vi "RichToFlatnixnet_grpc_ReadStateValue.vi"(5 "OutputClusterType":T1, 11 "InputCluster":T14) -> (3 "OutputCluster":T1)   [LabVIEW 2025, in "xnet-grpc_client.lvlib"]
uses:
  nixnet_grpc_ReadStateValue.ctl
  nixnet_grpc_ReadStateValue_value/nixnet_grpc_ReadStateValue_value.lvclass
  nixnet_grpc_ReadStateValue_Flat.ctl
  nixnet_grpc_CanCommResponse_Flat.ctl
  nixnet_grpc_CanCommState.ctl
  nixnet_grpc_CanLastErr.ctl
  nixnet_grpc_FlexRayCommResponse_Flat.ctl
  nixnet_grpc_FlexRayPocState.ctl
  nixnet_grpc_FlexRayStats_Flat.ctl
  nixnet_grpc_LinCommResponse_Flat.ctl
  nixnet_grpc_LinCommState.ctl
  nixnet_grpc_SessionInfoResponse_Flat.ctl
  nixnet_grpc_SessionInfoState.ctl
  nixnet_grpc_J1939CommState_Flat.ctl
  nixnet_grpc_TimeLocalNetwork_Flat.ctl
  xnet-grpc_client.lvlib
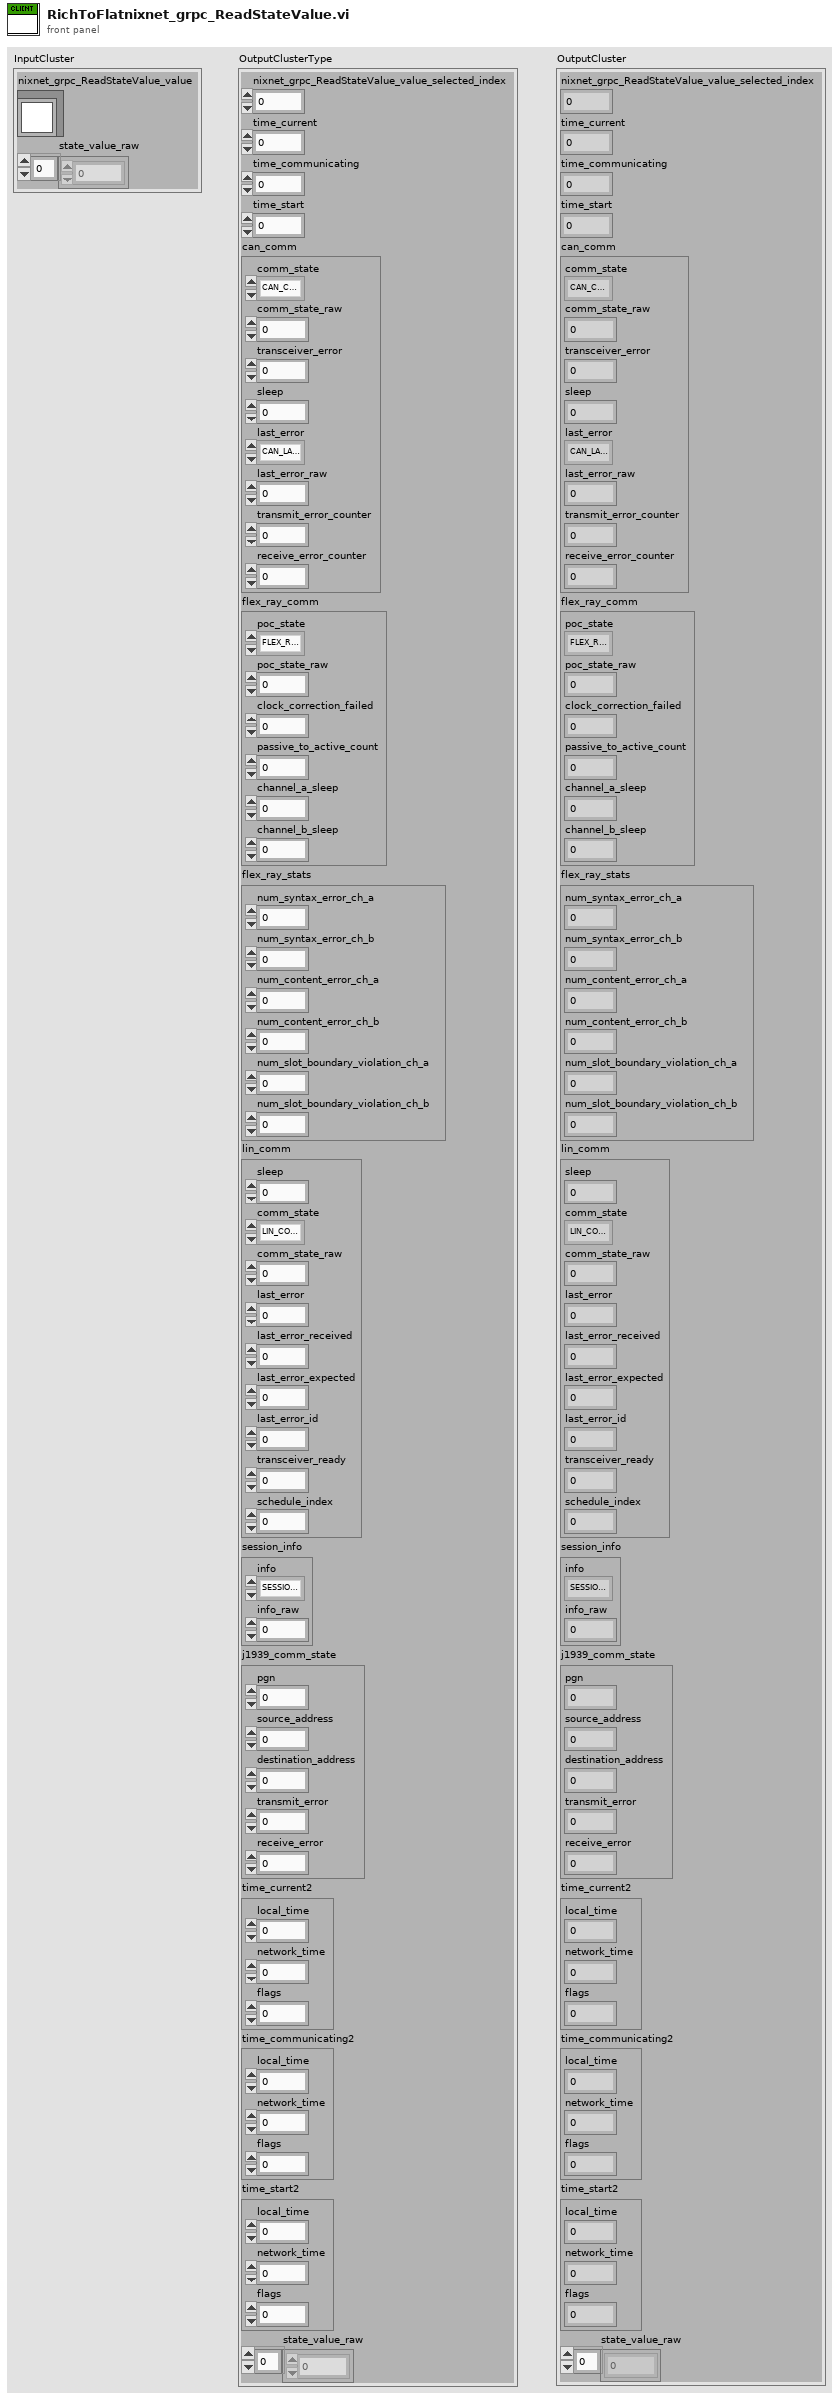
[diagram p1: front panel]
types:
  T1 = typedef "xnet-grpc_client.lvlib/nixnet_grpc_ReadStateValue_Flat.ctl" = cluster{"nixnet_grpc_ReadStateValue_value_selected_index":i32, "time_current":u64, "time_communicating":u64, "time_start":u64, "can_comm":T2, "flex_ray_comm":T5, "flex_ray_stats":T7, "lin_comm":T8, "session_info":T10, "j1939_comm_state":T12, "time_current2":T13, "time_communicating2":T13, "time_start2":T13, "state_value_raw":u8[]}
  T2 = typedef "xnet-grpc_client.lvlib/nixnet_grpc_CanCommResponse_Flat.ctl" = cluster{"comm_state":T3, "comm_state_raw":u32, "transceiver_error":u32, "sleep":u32, "last_error":T4, "last_error_raw":u32, "transmit_error_counter":u32, "receive_error_counter":u32}
  T3 = typedef "xnet-grpc_client.lvlib/nixnet_grpc_CanCommState.ctl" = enum32{"CAN_COMM_STATE_ERROR_ACTIVE", "CAN_COMM_STATE_ERROR_PASSIVE", "CAN_COMM_STATE_BUS_OFF", "CAN_COMM_STATE_INIT"}
  T4 = typedef "xnet-grpc_client.lvlib/nixnet_grpc_CanLastErr.ctl" = enum32{"CAN_LAST_ERR_NONE", "CAN_LAST_ERR_STUFF", "CAN_LAST_ERR_FORM", "CAN_LAST_ERR_ACK", "CAN_LAST_ERR_BIT_1", "CAN_LAST_ERR_BIT_0", "CAN_LAST_ERR_CRC"}
  T5 = typedef "xnet-grpc_client.lvlib/nixnet_grpc_FlexRayCommResponse_Flat.ctl" = cluster{"poc_state":T6, "poc_state_raw":u32, "clock_correction_failed":u32, "passive_to_active_count":u32, "channel_a_sleep":u32, "channel_b_sleep":u32}
  T6 = typedef "xnet-grpc_client.lvlib/nixnet_grpc_FlexRayPocState.ctl" = enum32{"FLEX_RAY_POC_STATE_DEFAULT_CONFIG", "FLEX_RAY_POC_STATE_READY", "FLEX_RAY_POC_STATE_NORMAL_ACTIVE", "FLEX_RAY_POC_STATE_NORMAL_PASSIVE", "FLEX_RAY_POC_STATE_HALT", "FLEX_RAY_POC_STATE_MONITOR", "FLEX_RAY_POC_STATE_CONFIG"}
  T7 = typedef "xnet-grpc_client.lvlib/nixnet_grpc_FlexRayStats_Flat.ctl" = cluster{"num_syntax_error_ch_a":u32, "num_syntax_error_ch_b":u32, "num_content_error_ch_a":u32, "num_content_error_ch_b":u32, "num_slot_boundary_violation_ch_a":u32, "num_slot_boundary_violation_ch_b":u32}
  T8 = typedef "xnet-grpc_client.lvlib/nixnet_grpc_LinCommResponse_Flat.ctl" = cluster{"sleep":u32, "comm_state":T9, "comm_state_raw":u32, "last_error":u32, "last_error_received":u32, "last_error_expected":u32, "last_error_id":u32, "transceiver_ready":u32, "schedule_index":u32}
  T9 = typedef "xnet-grpc_client.lvlib/nixnet_grpc_LinCommState.ctl" = enum32{"LIN_COMM_STATE_IDLE", "LIN_COMM_STATE_ACTIVE", "LIN_COMM_STATE_INACTIVE"}
  T10 = typedef "xnet-grpc_client.lvlib/nixnet_grpc_SessionInfoResponse_Flat.ctl" = cluster{"info":T11, "info_raw":u32}
  T11 = typedef "xnet-grpc_client.lvlib/nixnet_grpc_SessionInfoState.ctl" = enum32{"SESSION_INFO_STATE_STOPPED", "SESSION_INFO_STATE_STARTED", "SESSION_INFO_STATE_MIX"}
  T12 = typedef "xnet-grpc_client.lvlib/nixnet_grpc_J1939CommState_Flat.ctl" = cluster{"pgn":u32, "source_address":u32, "destination_address":u32, "transmit_error":u32, "receive_error":u32}
  T13 = typedef "xnet-grpc_client.lvlib/nixnet_grpc_TimeLocalNetwork_Flat.ctl" = cluster{"local_time":u64, "network_time":u64, "flags":u32}
  T14 = typedef "xnet-grpc_client.lvlib/nixnet_grpc_ReadStateValue.ctl" = cluster{"nixnet_grpc_ReadStateValue_value":refnum<class "nixnet_grpc_ReadStateValue_value.lvclass">, "state_value_raw":u8[]}
  T15 = typedef "xnet-grpc_client.lvlib/nixnet_grpc_CanCommResponse.ctl" = cluster{"comm_state":T3, "comm_state_raw":u32, "transceiver_error":u32, "sleep":u32, "last_error":T4, "last_error_raw":u32, "transmit_error_counter":u32, "receive_error_counter":u32}
  T16 = typedef "xnet-grpc_client.lvlib/nixnet_grpc_FlexRayCommResponse.ctl" = cluster{"poc_state":T6, "poc_state_raw":u32, "clock_correction_failed":u32, "passive_to_active_count":u32, "channel_a_sleep":u32, "channel_b_sleep":u32}
  T17 = typedef "xnet-grpc_client.lvlib/nixnet_grpc_FlexRayStats.ctl" = cluster{"num_syntax_error_ch_a":u32, "num_syntax_error_ch_b":u32, "num_content_error_ch_a":u32, "num_content_error_ch_b":u32, "num_slot_boundary_violation_ch_a":u32, "num_slot_boundary_violation_ch_b":u32}
  T18 = typedef "xnet-grpc_client.lvlib/nixnet_grpc_LinCommResponse.ctl" = cluster{"sleep":u32, "comm_state":T9, "comm_state_raw":u32, "last_error":u32, "last_error_received":u32, "last_error_expected":u32, "last_error_id":u32, "transceiver_ready":u32, "schedule_index":u32}
  T19 = typedef "xnet-grpc_client.lvlib/nixnet_grpc_SessionInfoResponse.ctl" = cluster{"info":T11, "info_raw":u32}
  T20 = typedef "xnet-grpc_client.lvlib/nixnet_grpc_J1939CommState.ctl" = cluster{"pgn":u32, "source_address":u32, "destination_address":u32, "transmit_error":u32, "receive_error":u32}
  T21 = typedef "xnet-grpc_client.lvlib/nixnet_grpc_TimeLocalNetwork.ctl" = cluster{"local_time":u64, "network_time":u64, "flags":u32}
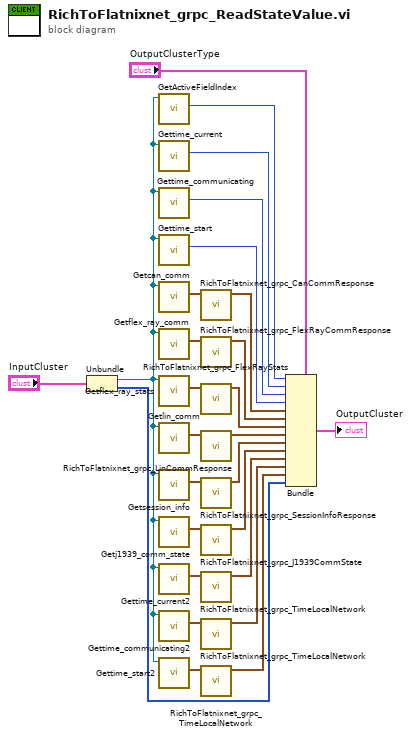
[diagram p0: block diagram]
diagram:
  n1 = Unbundle "Unbundle"("InputCluster") -> ("nixnet_grpc_ReadStateValue_value"=w24:refnum<class "nixnet_grpc_ReadStateValue_value.lvclass">, "state_value_raw"=w1:u8[])
  n2 = call "GetActiveFieldIndex.vi"("OneOfTemplate in"=w24) -> ("Active Field Index"=w23:i32)  [unwired: 8 in, 2 out]
  n3 = call "Gettime_current.vi"("OneOfTemplate in"=w24) -> ("Get_Val"=w22:u64)  [unwired: 8 in, 2 out]
  n4 = call "Gettime_communicating.vi"("OneOfTemplate in"=w24) -> ("Get_Val"=w21:u64)  [unwired: 8 in, 2 out]
  n5 = call "Gettime_start.vi"("OneOfTemplate in"=w24) -> ("Get_Val"=w20:u64)  [unwired: 8 in, 2 out]
  n6 = call "Getcan_comm.vi"("OneOfTemplate in"=w24) -> ("Get_Val"=w19:T15)  [unwired: 8 in, 2 out]
  n7 = call "Getflex_ray_comm.vi"("OneOfTemplate in"=w24) -> ("Get_Val"=w17:T16)  [unwired: 8 in, 2 out]
  n8 = call "Getflex_ray_stats.vi"("OneOfTemplate in"=w24) -> ("Get_Val"=w15:T17)  [unwired: 8 in, 2 out]
  n9 = call "Getlin_comm.vi"("OneOfTemplate in"=w24) -> ("Get_Val"=w13:T18)  [unwired: 8 in, 2 out]
  n10 = call "Getsession_info.vi"("OneOfTemplate in"=w24) -> ("Get_Val"=w11:T19)  [unwired: 8 in, 2 out]
  n11 = call "Getj1939_comm_state.vi"("OneOfTemplate in"=w24) -> ("Get_Val"=w9:T20)  [unwired: 8 in, 2 out]
  n12 = call "Gettime_current2.vi"("OneOfTemplate in"=w24) -> ("Get_Val"=w7:T21)  [unwired: 8 in, 2 out]
  n13 = call "Gettime_communicating2.vi"("OneOfTemplate in"=w24) -> ("Get_Val"=w5:T21)  [unwired: 8 in, 2 out]
  n14 = call "Gettime_start2.vi"("OneOfTemplate in"=w24) -> ("Get_Val"=w3:T21)  [unwired: 8 in, 2 out]
  n15 = call "RichToFlatnixnet_grpc_CanCommResponse.vi"("InputCluster"=w19) -> ("OutputCluster"=w18:T2)  [unwired: 10 in]
  n16 = call "RichToFlatnixnet_grpc_FlexRayCommResponse.vi"("InputCluster"=w17) -> ("OutputCluster"=w16:T5)  [unwired: 10 in]
  n17 = call "RichToFlatnixnet_grpc_FlexRayStats.vi"("InputCluster"=w15) -> ("OutputCluster"=w14:T7)  [unwired: 10 in]
  n18 = call "RichToFlatnixnet_grpc_LinCommResponse.vi"("InputCluster"=w13) -> ("OutputCluster"=w12:T8)  [unwired: 10 in]
  n19 = call "RichToFlatnixnet_grpc_SessionInfoResponse.vi"("InputCluster"=w11) -> ("OutputCluster"=w10:T10)  [unwired: 10 in]
  n20 = call "RichToFlatnixnet_grpc_J1939CommState.vi"("InputCluster"=w9) -> ("OutputCluster"=w8:T12)  [unwired: 10 in]
  n21 = call "RichToFlatnixnet_grpc_TimeLocalNetwork.vi"("InputCluster"=w7) -> ("OutputCluster"=w6:T13)  [unwired: 10 in]
  n22 = call "RichToFlatnixnet_grpc_TimeLocalNetwork.vi"("InputCluster"=w5) -> ("OutputCluster"=w4:T13)  [unwired: 10 in]
  n23 = call "RichToFlatnixnet_grpc_TimeLocalNetwork.vi"("InputCluster"=w3) -> ("OutputCluster"=w2:T13)  [unwired: 10 in]
  n24 = Bundle "Bundle"(cluster="OutputClusterType", "nixnet_grpc_ReadStateValue_value_selected_index"=w23, "time_current"=w22, "time_communicating"=w21, "time_start"=w20, "can_comm"=w18, "flex_ray_comm"=w16, "flex_ray_stats"=w14, "lin_comm"=w12, "session_info"=w10, "j1939_comm_state"=w8, "time_current2"=w6, "time_communicating2"=w4, "time_start2"=w2, "state_value_raw"=w1) -> (→"OutputCluster":T1)
